vi "IVCurveCustom.vi"(7 "OriginalSweepInfo":T1, 8 "ReadExtra":bool=TRUE, 9 "SweepInfo":T1, 10 "Program":string, 11 "UiDefinition":T4) -> (1 "appended array":dbl[][](array[numeric]), 3 "InfoCluster":T2)   [LabVIEW 2020]
uses:
  UIReferences.ctl
  C:/Users/User/Desktop/Automation/CurrentVersion/LabviewDXFViewer/bin/Release/LabviewDXFViewer.exe
  LabviewDXFViewer/bin/Release/LabviewDXFViewer.exe
  CapacitanceInfos.ctl
  CapacitanceRecord.ctl
  Keithley 2600 Series/Keithley 2600 Series.lvlib
panel:
  out "error out 4":errorcluster
  out "error out 3":errorcluster
  out "error out 2":errorcluster
  out "error out":errorcluster
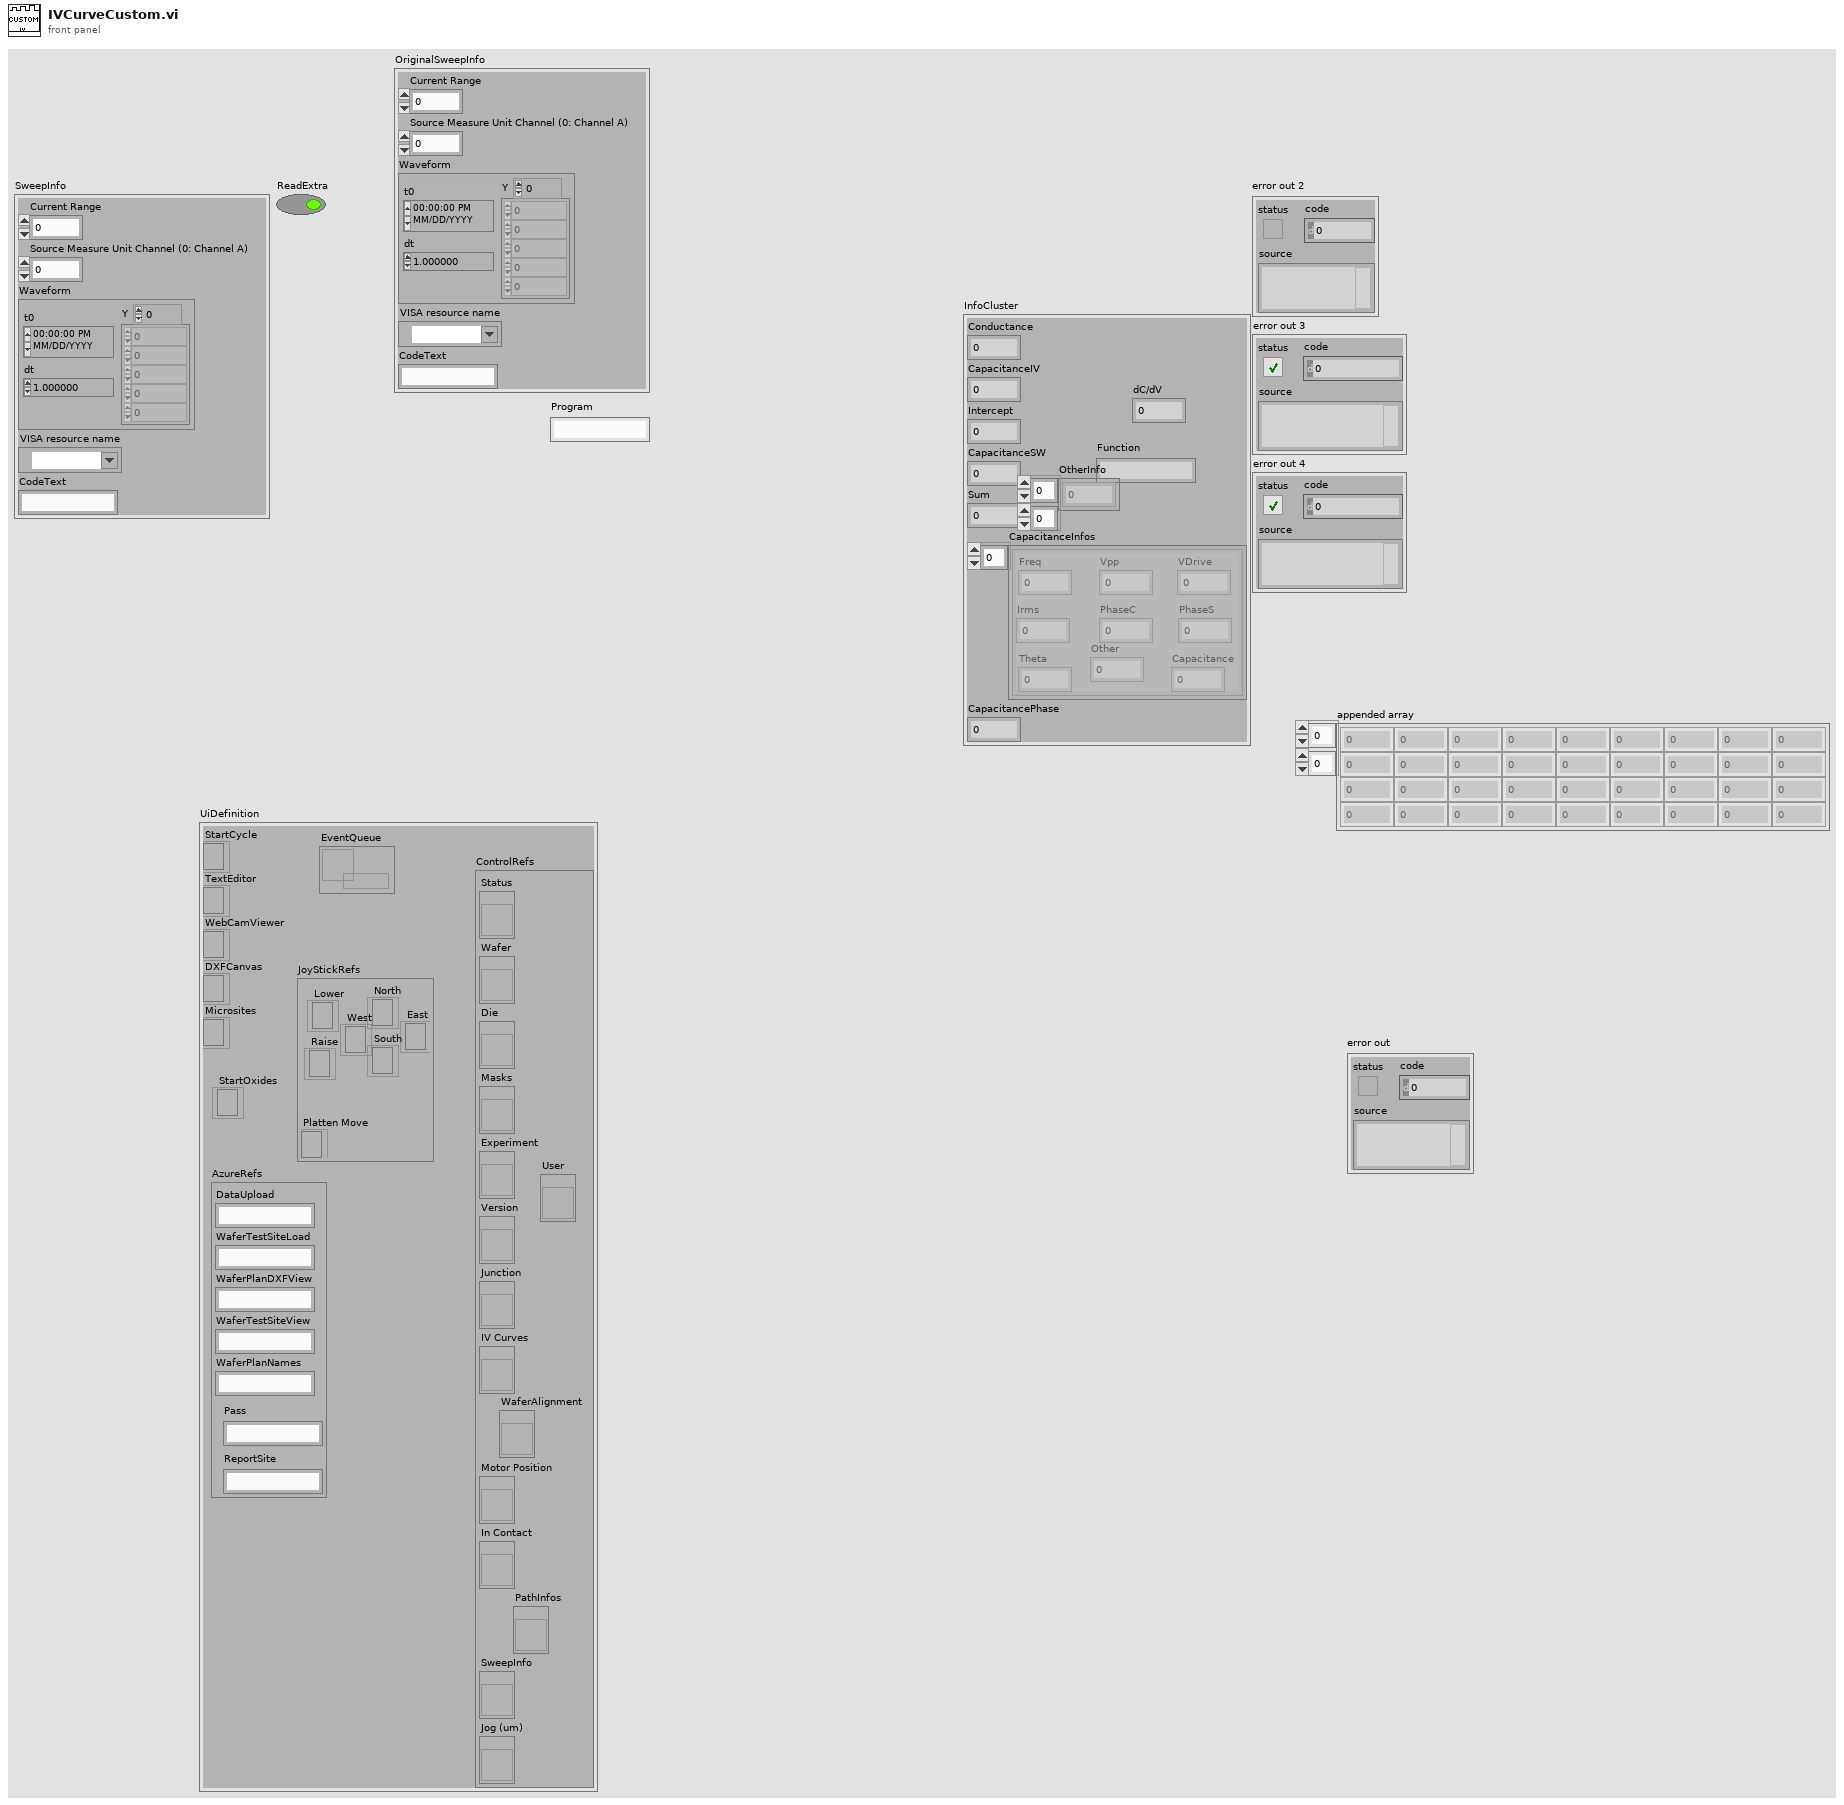
[diagram p1: front panel]
types:
  T1 = cluster{"Current Range":dbl, "Source Measure Unit Channel (0: Channel A)":i32, "Waveform":waveform(dbl), "VISA resource name":refnum<visa-resource-name>, "CodeText":string}
  T2 = typedef "CapacitanceInfos.ctl" = cluster{"Conductance":dbl, "CapacitanceIV":dbl, "Intercept":dbl, "CapacitanceSW":dbl, "Sum":dbl, "CapacitanceInfos":T3[], "CapacitancePhase":dbl, "dC/dV":dbl, "Function":string, "OtherInfo":dbl[][]}
  T3 = typedef "CapacitanceRecord.ctl" = cluster{"Freq":dbl, "Vpp":dbl, "PhaseS":dbl, "Irms":dbl, "PhaseC":dbl, "Theta":dbl, "VDrive":dbl, "Capacitance":dbl, "Other":dbl}
  T4 = typedef "UIReferences.ctl" = cluster{"StartCycle":refnum<k24>, "TextEditor":refnum<k24>, "WebCamViewer":refnum<k24>, "DXFCanvas":refnum<k24>, "Microsites":refnum<k24>, "JoyStickRefs":cluster{"North":refnum<k24>, "Lower":refnum<k24>, "Raise":refnum<k24>, "Platten Move":refnum<k24>, "West":refnum<k24>, "East":refnum<k24>, "South":refnum<k24>}, "AzureRefs":cluster{"DataUpload":string, "WaferTestSiteLoad":string, "WaferPlanDXFView":string, "WaferTestSiteView":string, "WaferPlanNames":string, "Pass":string, "ReportSite":string}, "ControlRefs":cluster{"Status":refnum<vi>, "Wafer":refnum<vi>, "Die":refnum<vi>, "Masks":refnum<vi>, "Experiment":refnum<vi>, "Version":refnum<vi>, "Junction":refnum<vi>, "IV Curves":refnum<vi>, "Motor Position":refnum<vi>, "In Contact":refnum<vi>, "SweepInfo":refnum<vi>, "Jog (um)":refnum<vi>, "PathInfos":refnum<vi>, "User":refnum<vi>, "WaferAlignment":refnum<vi>}, "EventQueue":refnum<queue>, "StartOxides":refnum<k24>}
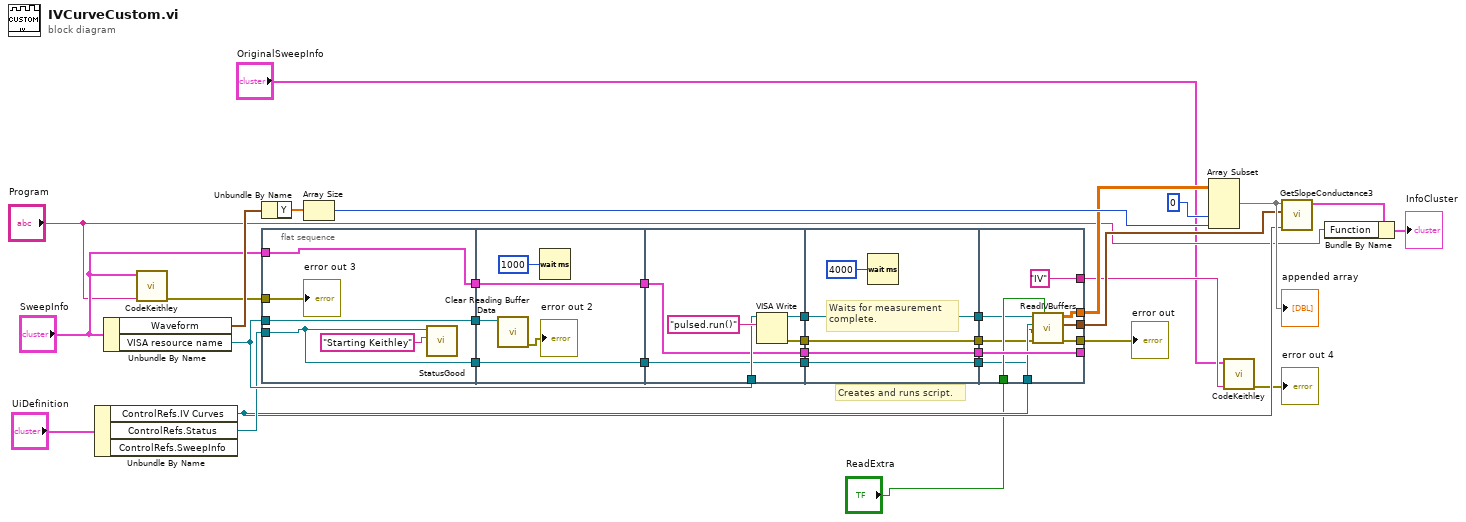
[diagram p0: block diagram]
diagram:
  # "Creates and runs script."
  n1 = Unbundle By Name("UiDefinition") -> ("ControlRefs.IV Curves"=w13:refnum<vi>, "ControlRefs.Status"=w25:refnum<vi>)  [unwired: 1 out]
  n2 = Unbundle By Name("SweepInfo") -> ("Waveform"=w31:waveform(dbl), "VISA resource name"=w32:refnum<visa-resource-name>)
  n3 = call "CodeKeithley.vi"("Program"="Program", "SweepInfo"="SweepInfo") -> ("error out"=w11:errorcluster)  [unwired: 9 in]
  n4 = Unbundle By Name(w31) -> ("Y"=w30:dbl[])
  n5 = flat-sequence {
    tunnel: w32 -> [w39]
    tunnel: [w39] -> w26
    tunnel: w25 -> [w35]
    tunnel: [w37] -> w24
    tunnel: "SweepInfo" -> [w37]
    tunnel: w11 -> [w36]
    tunnel: [w35] -> w4
    tunnel: w26 -> [w43]
    tunnel: w24 -> [w41]
    tunnel: [w41] -> w21
    tunnel: w4 -> [w40]
    tunnel: [w40] -> w3
    tunnel: [w48] -> w34
    tunnel: w32 -> [w49]
    tunnel: [w47] -> w22
    tunnel: w21 -> [w47]
    tunnel: [w46] -> w14
    tunnel: w3 -> [w45]
    tunnel: [w45] -> w2
    tunnel: w34 -> [w55]
    tunnel: w22 -> [w53]
    tunnel: [w55] -> w20
    tunnel: [w53] -> w19
    tunnel: [w52] -> w15
    tunnel: w14 -> [w52]
    tunnel: w2 -> [w51]
    tunnel: [w51] -> w1
    tunnel: [w65] -> _
    tunnel: w20 -> [w62]
    tunnel: w19 -> [w65]
    tunnel: "ReadExtra" -> [w64]
    tunnel: w13 -> [w63]
    tunnel: [w61] -> w18
    tunnel: [w60] -> w17
    tunnel: [w59] -> w16
    tunnel: w15 -> [w58]
    tunnel: ["IV" ("y")] -> w6
    tunnel: w1 -> [w56]
    frame #0 {
      n6 = call "StatusGood.vi"("Text.Text"="Starting Keithley", "String in"=w35) -> ()  [unwired: 10 in]
      "error out 3" <- w36
    }
    frame #1 {
      n7 = call "Clear Reading Buffer Data.vi"("VISA resource name"=w43) -> ("error out"=→"error out 2":errorcluster)  [unwired: 9 in, 1 out]
      n8 = Wait (ms)(milliseconds to wait=u32 1000) -> ()  [unwired: 1 out]
    }
    frame #2 {
      n9 = VISA Write(VISA resource name=w49, write buffer="pulsed.run()" ("format string")) -> (VISA resource name out=w48:refnum<visa-resource-name>, error out=w46:errorcluster)  [unwired: 1 in, 1 out]
    }
    frame #3 {
      # "Waits for measurement complete."
      n10 = Wait (ms)(milliseconds to wait=4000) -> ()  [unwired: 1 out]
    }
    frame #4 {
      n11 = call "ReadIVBuffers.vi"("GetCapacitors"=w64, "error in (no error)"=w58, "Status"=w56, "XYGraph Refnum"=w63, "VISA Refnum in"=w62) -> ("error out"=w61:errorcluster, "CapacitanceInfos"=w60:T3[], "Array"=w59:dbl[][])  [unwired: 4 in]
    }
  }
  n12 = Array Size(array=w30) -> (size(s)=w29:i32)
  n13 = Array Subset(array=w16, index (col)=0 ("index"), length (col)=w29) -> (w27:dbl[][])  [unwired: 2 in]
  "appended array" <- w27
  n14 = call "CodeKeithley.vi"("Program"=w6, "SweepInfo"="OriginalSweepInfo") -> ("error out"=→"error out 4":errorcluster)  [unwired: 9 in]
  n15 = call "GetSlopeConductance3.vi"("XYGraph Refnum"=w13, "CapacitanceRecords"=w17, "Array in"=w27) -> ("InfoCluster"=w10:T2)  [unwired: 7 in, 1 out]
  n16 = Bundle By Name(cluster=w10, "Function"="Program") -> (→"InfoCluster":T2)
  "error out" <- w18
